vi "Read PAR_index.vi"(11 "bronkhorst_reg in":refnum<class "bronkhorst_reg_2.lvclass">) -> (2 "PAR_indexes":i32[](array[numeric]), 3 "bronkhorst_reg out":refnum<class "bronkhorst_reg_2.lvclass">)   [LabVIEW 2019, in "control.lvlib" / "bronkhorst_reg_2.lvclass"]
uses:
  bronkhorst_reg_2.lvclass
  bronkhorst_reg_2.lvclass/bronkhorst_reg_2.ctl
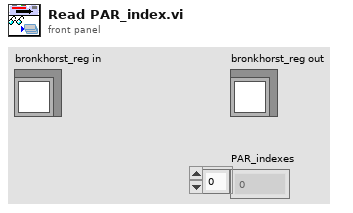
[diagram p1: front panel]
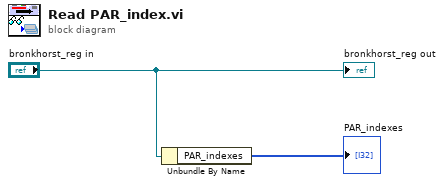
[diagram p0: block diagram]
diagram:
  n1 = Unbundle By Name("bronkhorst_reg in") -> ("PAR_indexes"=→"PAR_indexes":i32[])
  "bronkhorst_reg out" <- "bronkhorst_reg in"
